vi "ma_SML Linear Weighting.vi"   [LabVIEW 2020, in "NI_MAPro.lvlib"]
uses:
  NI_MAPro.lvlib
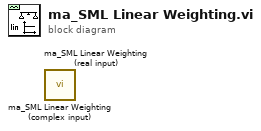
[diagram p0: block diagram]
diagram:
  n1 = call "ma_SML Linear Weighting (complex input).vi"() -> ()  [unwired: 3 in, 3 out]
  n2 = call "ma_SML Linear Weighting (real input).vi"() -> ()  [unwired: 3 in, 3 out]
